vi "Init Open Front Panel Tickbox.vi"(8 "Error In":errorcluster, 11 "\"Open Front Panel?\" Tickbox Ref":refnum<vi>) -> (0 "Error Out":errorcluster)   [LabVIEW 2022 SP3]
doc: "This VI initialises the \"Open Front Panel?\" tickbox.\n\nIt reads the setting value from the Windows Registry and sets the boolean value of the tickbox accordingly."
panel:
  # "Development\nControls or indicators that are useful for development or testing, but which are not outputs of the VI."
  # "Input\nInputs to the VI"
  # "Output\nOutputs of the VI"
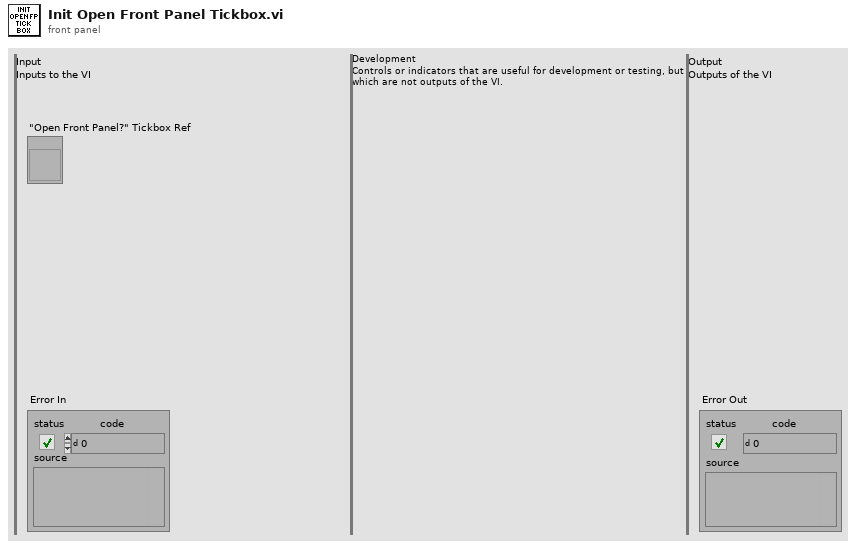
[diagram p1: front panel]
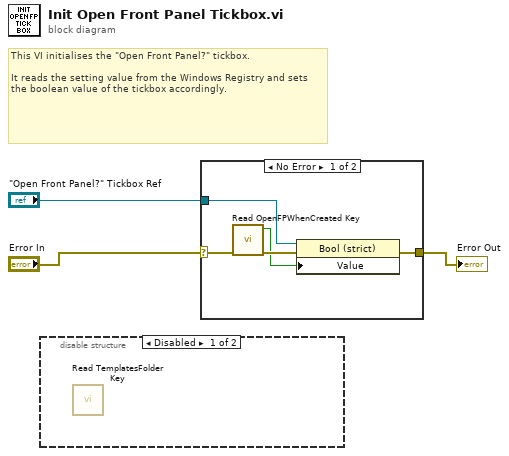
[diagram p0: block diagram]
diagram:
  # "This VI initialises the \"Open Front Panel?\" tickbox.\n\nIt reads the setting value from the Windows Registry and sets the boolean value of the tickbox accordingly."
  n1 = disable-structure shown="Disabled" {
    frame Disabled {
      n2 = call "Read TemplatesFolder Key.vi"() -> ()  [unwired: 10 in, 2 out]
    }
    frame Enabled {
    }
  }
  n3 = case shown="No Error" "Error In" {
    selector: "Error In" -> [w8 w9]
    tunnel: [w6 w9] -> w2
    tunnel: "\"Open Front Panel?\" Tickbox Ref" -> [w5 _]
    frame No Error {
      n4 = call "Read OpenFPWhenCreated Key.vi"("Error In"=w8) -> ("Error Out"=w7:errorcluster, "Open Front Panel When Created?"=w4:bool)  [unwired: 9 in]
      n5 = property class="Bool (strict)"(reference=w5, error in=w7, "Value"=w4) -> (error out=w6:errorcluster)  [unwired: 1 out]
    }
    frame Error {
    }
  }
  "Error Out" <- w2
